vi "Configure Measurement (Duty Cycle).vi"(7 "Duty Cycle Resolution (1)":dbl=1.0, 8 "error in (no error)":errorcluster, 9 "Frequency Estimate (10E+6 Hz)":dbl=10000000.0 format="%^#_6g", 10 "Channel (1:Channel 1)":i32(ring)=1 items=["Channel 1"=1, "Channel 2"=2], 11 "VISA resource name":refnum<visa-resource-name>) -> (0 "error out":errorcluster, 3 "VISA resource name out":refnum<visa-resource-name>)   [LabVIEW 2015, in "Template - Counter.lvlib"]
doc: "Configures the settings required for Duty Cycle measurements."
uses:
  <instrlib>/_Template - Counter/Template - Counter.lvlib
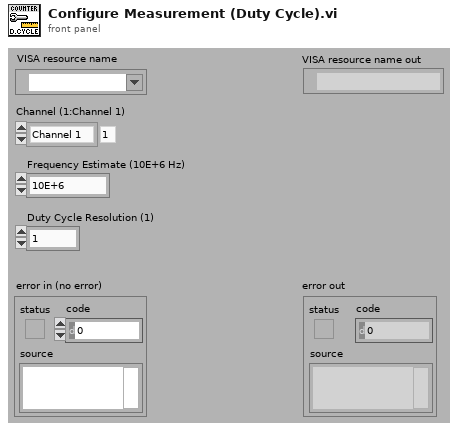
[diagram p1: front panel]
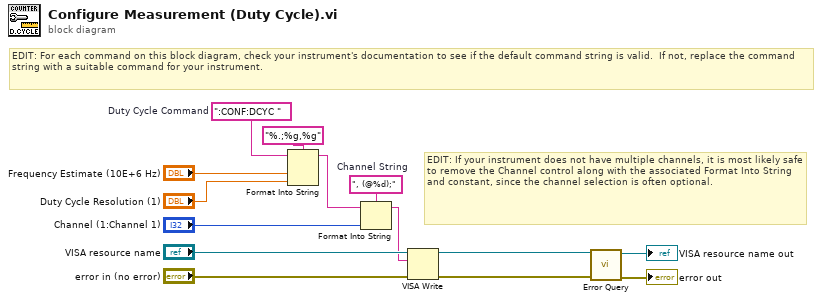
[diagram p0: block diagram]
diagram:
  w10 = ", (@%d);"  # Channel String
  w3 = ":CONF:DCYC "  # Duty Cycle Command
  # "EDIT: If your instrument does not have multiple channels, it is most likely safe to remove the Channel control along with the associated Format Into String and constant, since the channel selection is often optional."
  # "EDIT: For each command on this block diagram, check your instrument's documentation to see if the default command string is valid.  If not, replace the command string with a suitable command for your instrument."
  n1 = Format Into String(format string="%.;%g,%g", initial string=w3, "Frequency Estimate (10E+6 Hz)", "Duty Cycle Resolution (1)") -> (resulting string=w2:string)  [unwired: 1 in, 1 out]
  n2 = Format Into String(format string=w10, initial string=w2, "Channel (1:Channel 1)") -> (resulting string=w4:string)  [unwired: 1 in, 1 out]
  n3 = VISA Write(VISA resource name="VISA resource name", write buffer=w4, error in (no error)="error in (no error)") -> (VISA resource name out=w9:refnum<visa-resource-name>, error out=w7:errorcluster)  [unwired: 1 out]
  n4 = call <instrlib>:"Error Query.vi"("error in (no error)"=w7, "VISA resource name"=w9) -> ("error out"=→"error out":errorcluster, "VISA resource name out"=→"VISA resource name out":refnum<visa-resource-name>)  [unwired: 6 in, 2 out]
